vi "spi_clear.vi"(1 "address":u8, 2 "packet_id":u16) -> (0 "output cluster":T1 {"instruction" items=["default"=0, "write"=173, "read"=237, "clear"=205]; "data" format="%x"; "address" format="%x"})   [LabVIEW 2018]
uses:
  packet_t.ctl
  packet_type_t.ctl
  spi_instructions.ctl
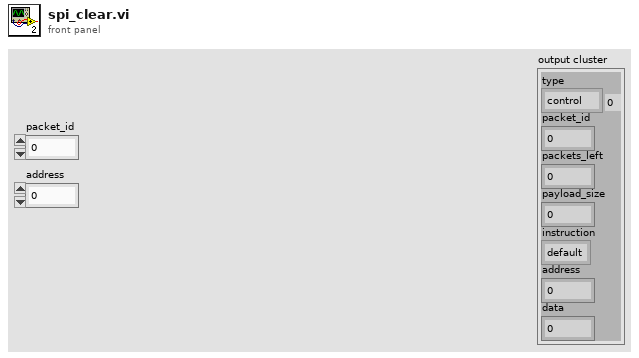
[diagram p1: front panel]
types:
  T1 = typedef "packet_t.ctl" = cluster{"type":T2, "packet_id":u16, "packets_left":u16, "payload_size":u16, "instruction":T3, "address":u8, "data":u8}
  T2 = typedef "packet_type_t.ctl" = enum8{"control", "spi", "audio", "hdmi"}
  T3 = typedef "spi_instructions.ctl" = u8
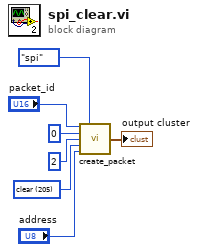
[diagram p0: block diagram]
diagram:
  w3 = T3 205 items=["default"=0, "write"=173, "read"=237, "clear"=205] ("instruction")
  n1 = call "create_packet.vi"("packet_id"="packet_id", "type"=packet_type_t."spi", "packets_left"=u16 0, "payload_size"=u16 2, "instruction"=w3, "address"="address") -> ("output cluster"=→"output cluster":T1)  [unwired: 9 in]
